vi "testDiagStackMat.vi"(8 "error in (no error)":errorcluster) -> (0 "error out":errorcluster)   [LabVIEW 2016]
doc: "Test to stack the matrixes (2D arrays actually) in the diagonal direction."
uses:
  <vilib>/addons/_JKI Toolkits/Caraya/classes/Assert/Assert.lvclass
  <vilib>/addons/_JKI Toolkits/Caraya/classes/Test/Test.lvclass
  MatOper/MatOper.lvclass
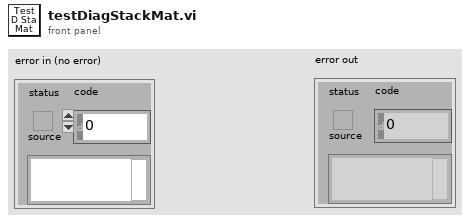
[diagram p1: front panel]
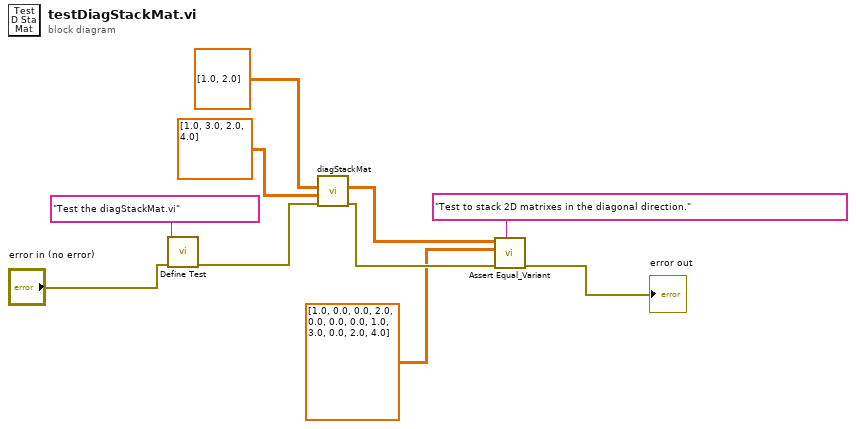
[diagram p0: block diagram]
diagram:
  n1 = call <vilib>:"Define Test.vi"("error in (no error)"="error in (no error)", "Label (VI Title)"="Test the diagStackMat.vi") -> ("error out"=w6:errorcluster)  [unwired: 9 in]
  n2 = call "diagStackMat.vi"("error in (no error)"=w6, "A1"=dbl[][] [[1.0, 3.0], [2.0, 4.0]], "A0"=dbl[][] [[1.0], [2.0]]) -> ("error out"=w5:errorcluster, "Diag Stack Matrix"=w2:dbl[][])  [unwired: 6 in, 1 out]
  n3 = call <vilib>:"Assert Equal_Variant.vi"("Label"="Test to stack 2D matrixes in the diagonal direction.", "error in (no error)"=w5, "Y"=dbl[][] [[1.0, 0.0, 0.0], [2.0, 0.0, 0.0], [0.0, 1.0, 3.0], [0.0, 2.0, 4.0]], "X"=w2) -> ("error out"=→"error out":errorcluster)  [unwired: 7 in]
